vi "instantiate_webpage_qa.vi"(0 "vectorestore":refnum<class "abstract_vector_base.lvclass">, 1 "skip_loading_data":bool, 5 "collection_name":string, 7 "chat_model":refnum<class "abstract_llm_base.lvclass">, 9 "embedding_model":refnum<class "abstract_llm_base.lvclass">, 11 "error in (no error)":errorcluster, 12 "webpages":string[](array[string])) -> (4 "agent_webpage_qa out":refnum<class "agent_webpage_qa.lvclass">, 15 "error out":errorcluster)   [LabVIEW 2020, in "agent_webpage_qa.lvclass"]
uses:
  agent_webpage_qa.lvclass
  D:/petwork/labview-llm-libraries/src/agent/agent_simple_qa/agent_simple_qa.lvclass
  models/abstract_llm_base/abstract_llm_base.lvclass
  vectorstore/abstract_vector_base/abstract_vector_base.lvclass
  data_source/datasource_webpage/datasource_webpage.lvclass
  D:/petwork/labview-llm-libraries/src/data_source/abstract_datasource_base/abstract_datasource_base.lvclass
  data_destination/destination_vectorstore/destination_vectorstore.lvclass
  D:/petwork/labview-llm-libraries/src/data_destination/abstract_datadestination_base/abstract_datadestination_base.lvclass
  data_processor/chunk_character_splitter/chunk_character_splitter.lvclass
  D:/petwork/labview-llm-libraries/src/data_processor/abstract_dataprocessing_base/abstract_dataprocessing_base.lvclass
  data_processor/embed_nodes/embed_nodes.lvclass
  data_pipeline/data_simple_pipeline/data_simple_pipeline.lvclass
  data_processor/abstract_dataprocessing_base/abstract_dataprocessing_base.lvclass
  agent_simple_qa/agent_simple_qa.lvclass
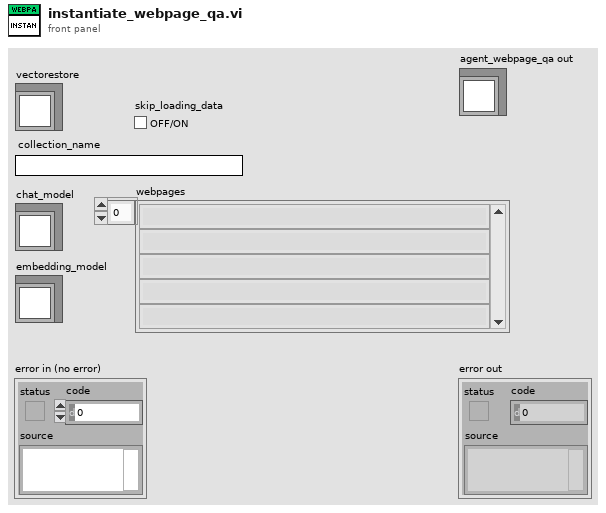
[diagram p1: front panel]
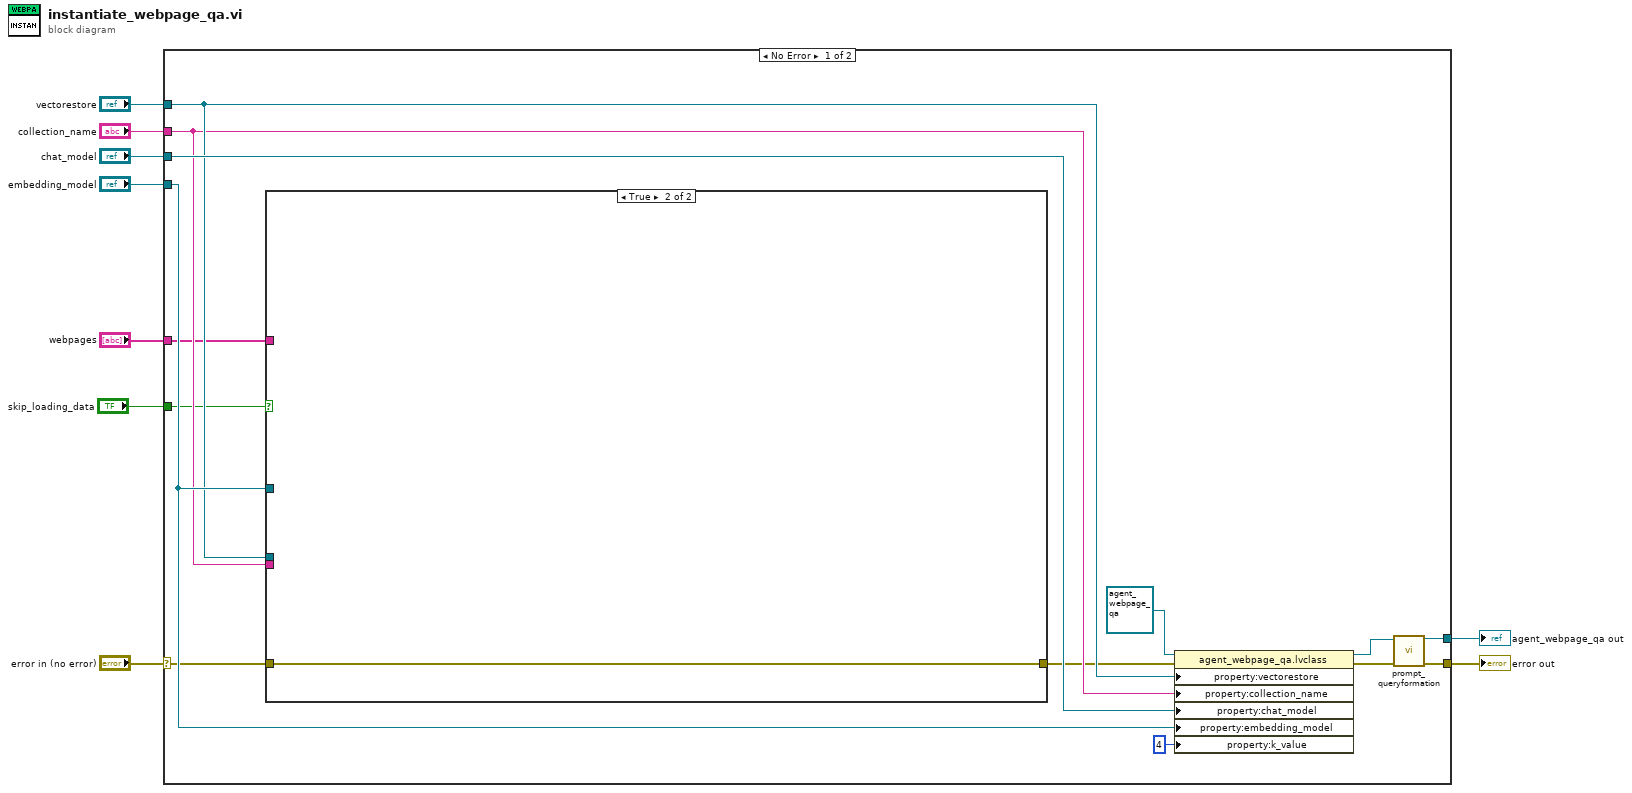
[diagram p0: block diagram]
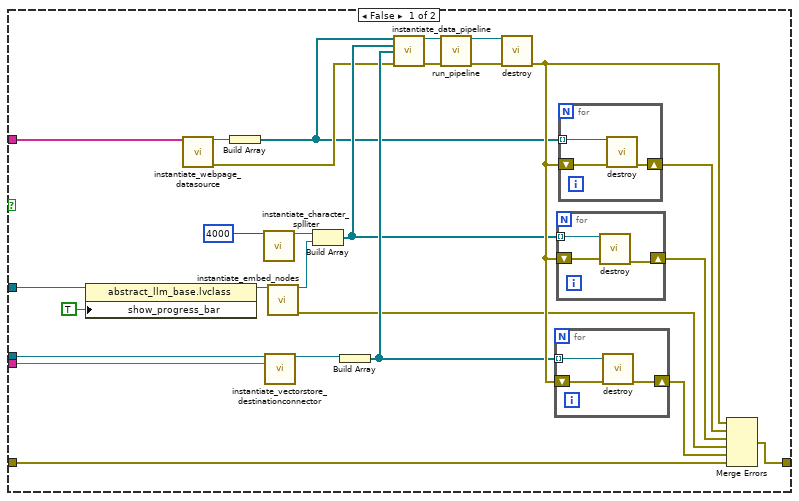
[diagram p2: hidden frame]
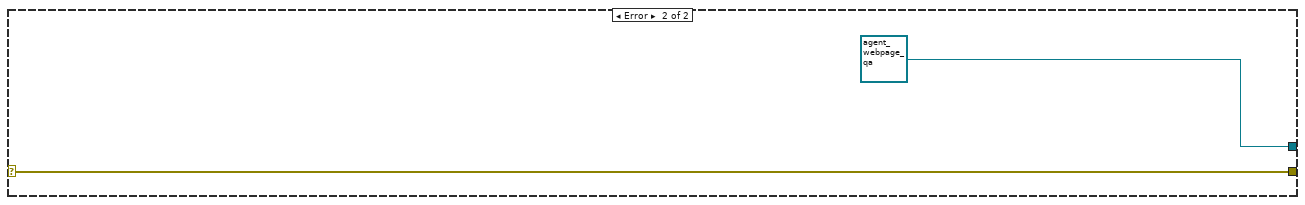
[diagram p3: hidden frame]
diagram:
  n1 = case shown="No Error" "error in (no error)" {
    selector: "error in (no error)" -> [w13 w61]
    tunnel: [w18 w61] -> w8
    tunnel: "vectorestore" -> [w15 _]
    tunnel: "collection_name" -> [w14 _]
    tunnel: "chat_model" -> [w22 _]
    tunnel: "embedding_model" -> [w16 _]
    tunnel: [w17 refnum<class "agent_webpage_qa.lvclass"> refnum ("agent_webpage_qa out")] -> w3
    tunnel: "webpages" -> [w11 _]
    tunnel: "skip_loading_data" -> [w10 _]
    frame No Error {
      n2 = case shown="True" w10 {
        tunnel: w16 -> [w33 _]
        tunnel: w15 -> [w30 _]
        tunnel: w14 -> [w29 _]
        tunnel: w13 -> [w28 w59]
        tunnel: [w27 w59] -> w12
        tunnel: w11 -> [w26 _]
        frame False {
          n3 = property class="abstract_llm_base.lvclass"(reference=w33, "show_progress_bar"=TRUE) -> (reference out=w25:refnum<class "abstract_llm_base.lvclass">)  [unwired: 1 in, 1 out]
          n4 = call "instantiate_webpage_datasource.vi"("webpages"=w26) -> ("datasource_webpage out"=w39:refnum<class "datasource_webpage.lvclass">, "error out"=w41:errorcluster)  [unwired: 13 in]
          n5 = Build Array(w39) -> (w40:refnum<class "datasource_webpage.lvclass">[])
          n6 = call "instantiate_character_splliter.vi"("max_character_length"=u32 4000) -> ("chunk_character_splitter out"=w42:refnum<class "chunk_character_splitter.lvclass">)  [unwired: 13 in, 1 out]
          n7 = call "instantiate_vectorstore_destinationconnector.vi"("abstract_vector_base"=w30, "store_id"=w29) -> ("destination_vectorstore out"=w46:refnum<class "destination_vectorstore.lvclass">)  [unwired: 12 in, 1 out]
          n8 = call "instantiate_embed_nodes.vi"("abstract_llm_embedding"=w25) -> ("embed_nodes out"=w43:refnum<class "embed_nodes.lvclass">, "error out"=w32:errorcluster)  [unwired: 13 in]
          n9 = Build Array(w42, w43) -> (w44:refnum<class "abstract_dataprocessing_base.lvclass">[])
          n10 = Build Array(w46) -> (w47:refnum<class "destination_vectorstore.lvclass">[])
          n11 = call "instantiate_data_pipeline.vi"("sources"=w40, "processing steps"=w44, "destinations"=w47, "error in (no error)"=w41) -> ("data_simple_pipeline out"=w35:refnum<class "data_simple_pipeline.lvclass">, "error out"=w36:errorcluster)  [unwired: 10 in]
          n12 = call-dynamic "run_pipeline.vi"("data_simple_pipeline in"=w35, "error in (no error)"=w36) -> ("data_simple_pipeline out"=w37:refnum<class "data_simple_pipeline.lvclass">, "error out"=w38:errorcluster)  [unwired: 12 in]
          n13 = call-dynamic "destroy.vi"("data_simple_pipeline in"=w37, "error in (no error)"=w38) -> ("error out"=w49:errorcluster)  [unwired: 12 in, 1 out]
          n14 = for {
            shift-right: [w52] -> w31
            shift-left: w49 -> [w51]
            tunnel: w47 -> [w50] mode=indexing
            n15 = call-dynamic "destroy.vi"("abstract_datadestination_base in"=w50, "error in (no error)"=w51) -> ("error out"=w52:errorcluster)  [unwired: 12 in, 1 out]
          }
          n16 = for {
            tunnel: w44 -> [w55] mode=indexing
            shift-right: [w53] -> w45
            shift-left: w49 -> [w54]
            n17 = call-dynamic "destroy.vi"("abstract_dataprocessing_base in"=w55, "error in (no error)"=w54) -> ("error out"=w53:errorcluster)  [unwired: 12 in, 1 out]
          }
          n18 = for {
            tunnel: w40 -> [w58] mode=indexing
            shift-right: [w56] -> w48
            shift-left: w49 -> [w57]
            n19 = call-dynamic "destroy.vi"("abstract_datasource_base in"=w58, "error in (no error)"=w57) -> ("error out"=w56:errorcluster)  [unwired: 12 in, 1 out]
          }
          n20 = Merge Errors(w49, w48, w45, w32, w31, w28) -> (w27:errorcluster)
        }
        frame True {
        }
      }
      n21 = property class="agent_webpage_qa.lvclass"(reference=refnum<class "agent_webpage_qa.lvclass"> refnum ("agent_webpage_qa out"), error in=w12, "property:vectorestore"=w15, "property:collection_name"=w14, "property:chat_model"=w22, "property:embedding_model"=w16, "property:k_value"=u32 4 ("k_value")) -> (reference out=w19:refnum<class "agent_webpage_qa.lvclass">, error out=w20:errorcluster)
      n22 = call "prompt_queryformation.vi"("error in (no error)"=w20, "agent_simple_qa in"=w19) -> ("error out"=w18:errorcluster, "agent_simple_qa out"=w17:refnum<class "agent_webpage_qa.lvclass">)  [unwired: 8 in]
    }
    frame Error {
    }
  }
  "error out" <- w8
  "agent_webpage_qa out" <- w3
